vi "TryUpdateInclinometerSample.vi"   [LabVIEW 2016]
uses:
  <vilib>/Platform/TimedLoop/XDataNode/timing_clust.ctl
  <vilib>/Platform/TimedLoop/XDataNode/nitl_modes.ctl
  <vilib>/Platform/TimedLoop/XDataNode/wakeup.ctl
  Telemetry/TelemetryDataTypes.ctl
  Telemetry/TelemetryUpdateModes.ctl
  Telemetry/TelemetryFields.ctl
  <vilib>/rvi/Emulation/niFpgaEmulationIsFPGAContextNoSignature.vi
  <vilib>/rvi/Emulation/niFpgaSctlEmulationGetInTimedLoop.vi
  <vilib>/rvi/errors/niFpgaSetErrorForExecOnDevCompSimple.vi
  <vilib>/rvi/eio/common/nirviEmuReportErrorAndStop.vi
  <vilib>/rvi/DataTransferAndStorage/Container/Common/niFpgaContainerGetUniqueNameForEmu.vi
  <vilib>/rvi/FIFO/Fifo_Resource/nirvififoEmulationSetSize.vi
  <vilib>/rvi/FIFO/Fifo_Resource/nirviFifoEmulationQueueMgr.vi
  <instcachedir>/0/nirviFifoEmulationQueueMgr_E5CAEC123FF24DC58D834DCA3CDAA9B5.lvgen/nirviFifoEmulationQueueMgr_E5CAEC123FF24DC58D834DCA3CDAA9B5_035.vi
  <vilib>/Utility/error.llb/Clear Errors.vi
  <vilib>/rvi/FIFO/Fifo_Resource/nirvififoEmulationCreateLock.vi
  <vilib>/rvi/Emulation/niFpgaProcessEmulError.vi
  <vilib>/rvi/FIFO/Fifo_Resource/nirvififoEmulationObtainLock.vi
  <vilib>/rvi/FIFO/Fifo_Resource/nirvififoEmulationReleaseLock.vi
  <vilib>/rvi/occurrence/nirviWaitOnOccurrenceBase.vi
  <vilib>/rvi/errors/nirviReportUnexpectedCaseInternalError.vi
  <vilib>/rvi/errors/nirviReportUnexpectedCaseInternalError (U32).vi
  <vilib>/rvi/Emulation/niFpgaEmulationReportErrorSimple.vi
  <vilib>/rvi/Emulation/niFpgaGetClockAttributes.vi
  <vilib>/rvi/Emulation/niFpgaCriticalErrorInLSC.vi
  <instcachedir>/0/nirviFifoEmulationQueueMgr_E5CAEC123FF24DC58D834DCA3CDAA9B5.lvgen/nirviFifoEmulationQueueMgr_E5CAEC123FF24DC58D834DCA3CDAA9B5_038.vi
  <vilib>/rvi/FIFO/Fifo_Resource/nirvififoEmulationDetermineInputValidOut.vi
  <instcachedir>/0/nirviFifoEmulationQueueMgr_E5CAEC123FF24DC58D834DCA3CDAA9B5.lvgen/nirviFifoEmulationQueueMgr_E5CAEC123FF24DC58D834DCA3CDAA9B5_039.vi
  <vilib>/rvi/Memory/Memory_Emulation/niFpgaMemoryEmulationCacheClearOnFirstRun.vi
  <vilib>/rvi/Memory/Memory_Emulation/nirvimemoryEmulationManagerCache_MakeExclusive.vi
  <vilib>/rvi/Memory/Memory_Emulation/niFpgaMemoryEmulationValidateCache.vi
  <vilib>/rvi/Memory/Memory_Emulation/nirvimemoryEmulationManagerCache_InsertValue.vi
  <vilib>/rvi/Memory/Memory_Emulation/nirvimemoryEmulationManagerCache_ReleaseExclusive.vi
  <vilib>/rvi/Memory/Memory_Emulation/nirvimemoryEmulationManagerCache_GetValue.vi
  <vilib>/rvi/Memory/Memory_Emulation/nirvimemoryEmulationManagerCache_SetValue.vi
  <instcachedir>/0/nirviFifoEmulationQueueMgr_E5CAEC123FF24DC58D834DCA3CDAA9B5.lvgen/nirviFifoEmulationQueueMgr_E5CAEC123FF24DC58D834DCA3CDAA9B5_004.vi
  <vilib>/rvi/DataTransferAndStorage/Container/XNode/niFpgaContainer.xnode
  <vilib>/rvi/FIFO/Fifo_Resource/nirvififoEmulationRead.vi
  <vilib>/Platform/TimedLoop/XDataNode/XDataNode.xnode
  <vilib>/rvi/FIFO/Fifo_Resource/nirvififoEmulationWrite.vi
  <vilib>/rvi/DataTransferAndStorage/Register/Emulation/niFpgaRegisterEmulation.vi
  <vilib>/Platform/TimedLoop/XDataNode/XDNodeRunTimeDep.lvlib
types:
  T1 = cluster{"Timestamp":u64, "TxBytes":u64, "RxBytes":u64, "TxFrames":u64, "RxFrames":u64, "RawAngle":i32, "ZenithAngle":sgl}
  T2 = typedef "TelemetryFields.ctl" = enum16{"None", "InclinometerTxBytes", "InclinometerRxBytes", "InclinometerTxFrames", "InclinometerRxFrames", "InclinometerErrorTimestamp", "InclinometerErrorCode", "InclinometerSampleTimestamp", "InclinometerRawAngle", "InclinometerZenithAngle", "DisplacementTxBytes", "DisplacementRxBytes", "DisplacementTxFrames", "DisplacementRxFrames", "DisplacementErrorTimestamp", "DisplacementErrorCode", "DisplacementSampleTimestamp", "DisplacementRaw1", "DisplacementRaw2", "DisplacementRaw3", "DisplacementRaw4", "DisplacementRaw5", "DisplacementRaw6", "DisplacementRaw7", "DisplacementRaw8", "DisplacementEng1", "DisplacementEng2", "DisplacementEng3", "DisplacementEng4", "DisplacementEng5", "DisplacementEng6", "DisplacementEng7", "DisplacementEng8", "DisplacementPositionX", "DisplacementPositionY", "DisplacementPositionZ", "DisplacementRotationX", "DisplacementRotationY", "DisplacementRotationZ", "AccelerometerSampleCount", "AccelerometerSampleTimestamp", "AccelerometerRaw1", "AccelerometerRaw2", "AccelerometerRaw3", "AccelerometerRaw4", "AccelerometerRaw5", "AccelerometerRaw6", "AccelerometerRaw7", "AccelerometerRaw8", "AccelerometerEng1", "AccelerometerEng2", "AccelerometerEng3", "AccelerometerEng4", "AccelerometerEng5", "AccelerometerEng6", "AccelerometerEng7", "AccelerometerEng8", "AngularAccelerationX", "AngularAccelerationY", "AngularAccelerationZ", "GyroTxBytes", "GyroRxBytes", "GyroTxFrames", "GyroRxFrames", "GyroErrorTimestamp", "GyroErrorCode", "GyroSampleTimestamp", "AngularVelocityX", "AngularVelocityY", "AngularVelocityZ", "GyroStatus", "GyroSequenceNumber", "GyroTemperature", "GyroBITTimestamp", "GyroBIT0", "GyroBIT1", "GyroBIT2", "GyroBIT3", "GyroBIT4", "GyroBIT5", "GyroBIT6", "GyroBIT7"}
  T3 = typedef "TelemetryUpdateModes.ctl" = enum8{"=", "+", "-", "|"}
  T4 = typedef "TelemetryDataTypes.ctl" = enum8{"U8", "U16", "U32", "U64", "I8", "I16", "I32", "I64", "SGL"}
  T5 = typedef "XDNodeRunTimeDep.lvlib/timing_clust.ctl" = cluster{"Expected End [f-1]":u64, "Actual End [f-1]":u64, "Finished Late? [f-1]":bool, "Expected End [i-1]":u64, "Actual End [i-1]":u64, "Finished Late? [i-1]":bool, "Expected Start [i]":u64, "Actual Start [i]":u64, "Expected Start [f]":u64, "Actual Start [f]":u64, "Source Name":string, "Structure Name":string, "Period":i64, "Deadline":i64, "Offset":i64, "Start":i64, "Priority":i32, "Timeout":i32, "Mode":T6, "Wakeup Reason":T7, "Error":errorcluster, "Source Type":string, "Secondary Source Type":string, "Global End Time":u64, "Global Start Time":u64, "Frame Duration":u64, "Iteration Duration":u64, "Assigned CPU":i32, "I/O Scan Engine Mode":u32}
  T6 = typedef "XDNodeRunTimeDep.lvlib/nitl_modes.ctl" = enum32{"No Change", "Process missed periods, maintain original phase", "Discard missed periods, maintain original phase", "Process missed periods, ignore original phase", "Discard missed periods, ignore original phase"}
  T7 = typedef "XDNodeRunTimeDep.lvlib/wakeup.ctl" = enum32{"Normal", "Aborted", "Asynchronous wakeup", "Timing source error", "Timed loop error", "Timeout"}
  T8 = typedef "TelemetryUpdateData.ctl" = cluster{"DataType":T4, "Mode":T3, "Field":T2, "Data":u64}
  T9 = typedef "TelemetryUpdateDataSGL.ctl" = cluster{"Mode":T3, "Field":T2, "Data":sgl}
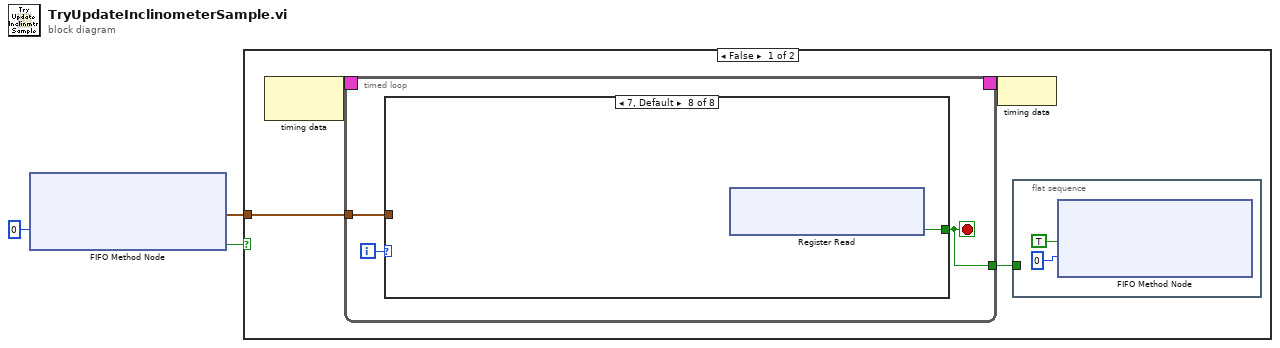
[diagram p0: block diagram]
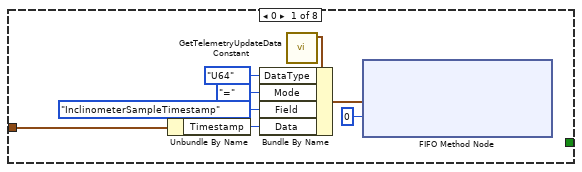
[diagram p2: hidden frame]
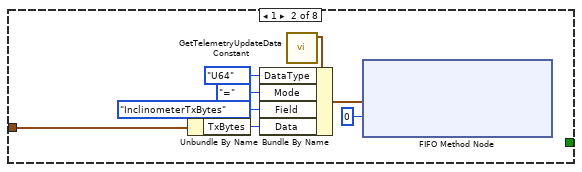
[diagram p3: hidden frame]
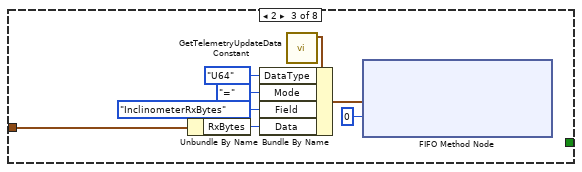
[diagram p4: hidden frame]
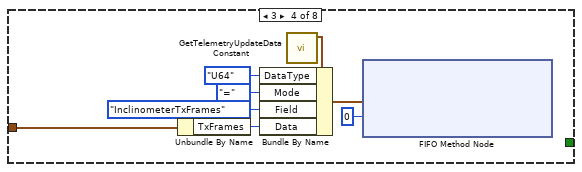
[diagram p5: hidden frame]
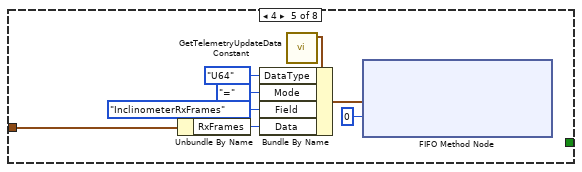
[diagram p6: hidden frame]
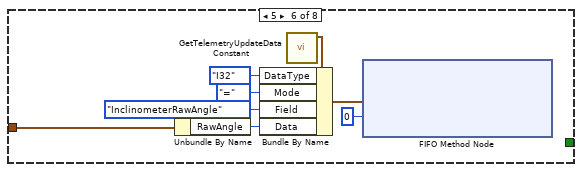
[diagram p7: hidden frame]
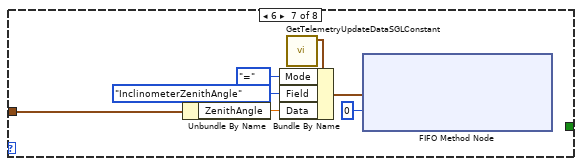
[diagram p8: hidden frame]
diagram:
  n1 = xnode ("FIFO Method Node")("Timeout"=0) -> ("Element"=w1:T1, "Timed Out?"=w2:bool)  [unwired: 1 in, 1 out]
  n2 = case shown="False" w2 {
    tunnel: w1 -> [w7 _]
    frame False {
      n3 = node-c288() -> (w6:T5)  [unwired: 1 in]
      n4 = timed-loop {
        tunnel: w7 -> [w10]
        timing: w6 -> [_]
        timing-out: [_] -> w5
        tunnel: [w8] -> w4
        i -> [w9]
        stop <- w8 stop-if-true
        n5 = case shown="7, Default" w9 {
          tunnel: [_ _ _ _ _ _ _ w66] -> w8
          tunnel: w10 -> [w11 w19 w27 w35 w44 w51 w59 _]
          frame 0 {
            n6 = Unbundle By Name(w11) -> ("Timestamp"=w17:u64)
            n7 = call "GetTelemetryUpdateDataConstant.vi"() -> ("TelemetryUpdateData"=w16:T8)  [unwired: 11 in]
            n8 = Bundle By Name(cluster=w16, "DataType"=TelemetryDataTypes."U64", "Mode"=TelemetryUpdateModes."=", "Field"=TelemetryFields."InclinometerSampleTimestamp" ("TelemetryFields"), "Data"=w17) -> (w13:T8)
            n9 = xnode ("FIFO Method Node")("Element"=w13, "Timeout"=0) -> ()  [unwired: 1 in, 2 out]
          }
          frame 1 {
            n10 = Unbundle By Name(w19) -> ("TxBytes"=w20:u64)
            n11 = call "GetTelemetryUpdateDataConstant.vi"() -> ("TelemetryUpdateData"=w21:T8)  [unwired: 11 in]
            n12 = Bundle By Name(cluster=w21, "DataType"=TelemetryDataTypes."U64", "Mode"=TelemetryUpdateModes."=", "Field"=TelemetryFields."InclinometerTxBytes", "Data"=w20) -> (w25:T8)
            n13 = xnode ("FIFO Method Node")("Element"=w25, "Timeout"=0) -> ()  [unwired: 1 in, 2 out]
          }
          frame 2 {
            n14 = Unbundle By Name(w27) -> ("RxBytes"=w34:u64)
            n15 = call "GetTelemetryUpdateDataConstant.vi"() -> ("TelemetryUpdateData"=w33:T8)  [unwired: 11 in]
            n16 = Bundle By Name(cluster=w33, "DataType"=TelemetryDataTypes."U64", "Mode"=TelemetryUpdateModes."=", "Field"=TelemetryFields."InclinometerRxBytes", "Data"=w34) -> (w29:T8)
            n17 = xnode ("FIFO Method Node")("Element"=w29, "Timeout"=0) -> ()  [unwired: 1 in, 2 out]
          }
          frame 3 {
            n18 = Unbundle By Name(w35) -> ("TxFrames"=w36:u64)
            n19 = call "GetTelemetryUpdateDataConstant.vi"() -> ("TelemetryUpdateData"=w37:T8)  [unwired: 11 in]
            n20 = Bundle By Name(cluster=w37, "DataType"=TelemetryDataTypes."U64", "Mode"=TelemetryUpdateModes."=", "Field"=TelemetryFields."InclinometerTxFrames", "Data"=w36) -> (w41:T8)
            n21 = xnode ("FIFO Method Node")("Element"=w41, "Timeout"=0) -> ()  [unwired: 1 in, 2 out]
          }
          frame 4 {
            n22 = Unbundle By Name(w44) -> ("RxFrames"=w43:u64)
            n23 = call "GetTelemetryUpdateDataConstant.vi"() -> ("TelemetryUpdateData"=w50:T8)  [unwired: 11 in]
            n24 = Bundle By Name(cluster=w50, "DataType"=TelemetryDataTypes."U64", "Mode"=TelemetryUpdateModes."=", "Field"=TelemetryFields."InclinometerRxFrames", "Data"=w43) -> (w46:T8)
            n25 = xnode ("FIFO Method Node")("Element"=w46, "Timeout"=0) -> ()  [unwired: 1 in, 2 out]
          }
          frame 5 {
            n26 = Unbundle By Name(w51) -> ("RawAngle"=w52:i32)
            n27 = call "GetTelemetryUpdateDataConstant.vi"() -> ("TelemetryUpdateData"=w53:T8)  [unwired: 11 in]
            n28 = Bundle By Name(cluster=w53, "DataType"=TelemetryDataTypes."I32", "Mode"=TelemetryUpdateModes."=", "Field"=TelemetryFields."InclinometerRawAngle" ("TelemetryFields"), "Data"=w52) -> (w56:T8)
            n29 = xnode ("FIFO Method Node")("Element"=w56, "Timeout"=0) -> ()  [unwired: 1 in, 2 out]
          }
          frame 6 {
            n30 = Unbundle By Name(w59) -> ("ZenithAngle"=w65:sgl)
            n31 = call "GetTelemetryUpdateDataSGLConstant.vi"() -> ("TelemetryUpdateDataSGL"=w60:T9)  [unwired: 11 in]
            n32 = Bundle By Name(cluster=w60, "Mode"=TelemetryUpdateModes."=", "Field"=TelemetryFields."InclinometerZenithAngle", "Data"=w65) -> (w61:T9)
            n33 = xnode ("FIFO Method Node")("Element"=w61, "Timeout"=0) -> ()  [unwired: 1 in, 2 out]
          }
          frame 7, Default {
            n34 = xnode ("Register Read")() -> ("Data"=w66:bool)  [unwired: 1 in, 1 out]
          }
        }
      }
      n35 = node-c288(w5) -> ()
      n36 = flat-sequence {
        tunnel: w4 -> [_]
        frame #0 {
          n37 = xnode ("FIFO Method Node")("Element"=TRUE, "Timeout"=0) -> ()  [unwired: 1 in, 2 out]
        }
      }
    }
    frame True {
    }
  }
